vi "CAlex2_SetCuff_Thigh_Treadmill.vi"(9 "Extra Weight (kg)":dbl, 10 "Upper Cuff to Lower Cuff (m)":dbl, 11 "Lower Cuff to Knee (m)":dbl) -> (2 "Thigh Cuff Low":T1={"BodyID"=0, "CoM(CuffCS)"={"Coord4"=[0.0, 0.0, 0.0, 1.0], "ID"=0}, "Mass(kg)"=0.0, "CablePts(CuffCS)"=[], "Cuff->Body"=[[1.0, 0.0, 0.0, 0.0], [0.0, 1.0, 0.0, 0.0], [0.0, 0.0, 1.0, 0.0], [0.0, 0.0, 0.0, 1.0]]}, 3 "Thigh Cuff High":T1={"BodyID"=0, "CoM(CuffCS)"={"Coord4"=[0.0, 0.0, 0.0, 1.0], "ID"=0}, "Mass(kg)"=0.0, "CablePts(CuffCS)"=[], "Cuff->Body"=[[1.0, 0.0, 0.0, 0.0], [0.0, 1.0, 0.0, 0.0], [0.0, 0.0, 1.0, 0.0], [0.0, 0.0, 0.0, 1.0]]})   [LabVIEW 2016, in "CAlex2.lvclass"]
uses:
  CAlex2.lvclass
  SerialChain-Cable/TypeDef/Cuff.ctl
  SerialChain/TypeDef/PointOnBody.ctl
  <vilib>/Analysis/Matrix/Datatypes/RealMatrix.ctl
  SerialChain/TypeDef/xyzO.ctl
  <vilib>/Analysis/Matrix/NI_Matrix.lvlib
  SerialChain/SerialChain.lvclass
  SerialChain-Cable/SerialChain-Cable.lvclass
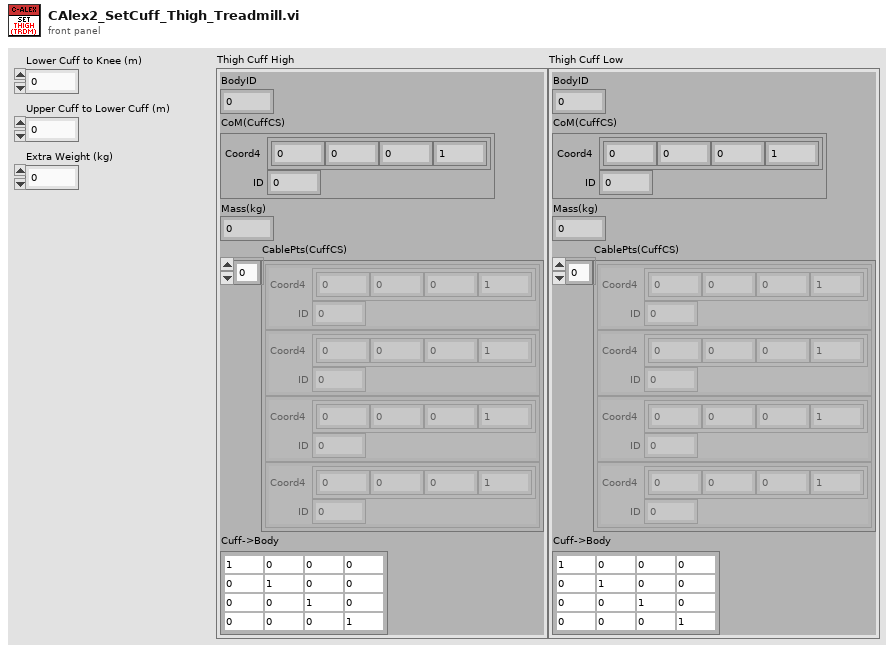
[diagram p1: front panel]
types:
  T1 = typedef "SerialChain-Cable.lvclass/Cuff.ctl" = cluster{"BodyID":i32, "CoM(CuffCS)":T2, "Mass(kg)":dbl, "CablePts(CuffCS)":T2[], "Cuff->Body":T3}
  T2 = typedef "SerialChain.lvclass/PointOnBody.ctl" = cluster{"Coord4":dbl[], "ID":i32}
  T3 = typedef "NI_Matrix.lvlib/RealMatrix.ctl" = dbl[][]
  T4 = typedef "SerialChain.lvclass/xyzO.ctl" = enum16{"X", "Y", "Z", "O"}
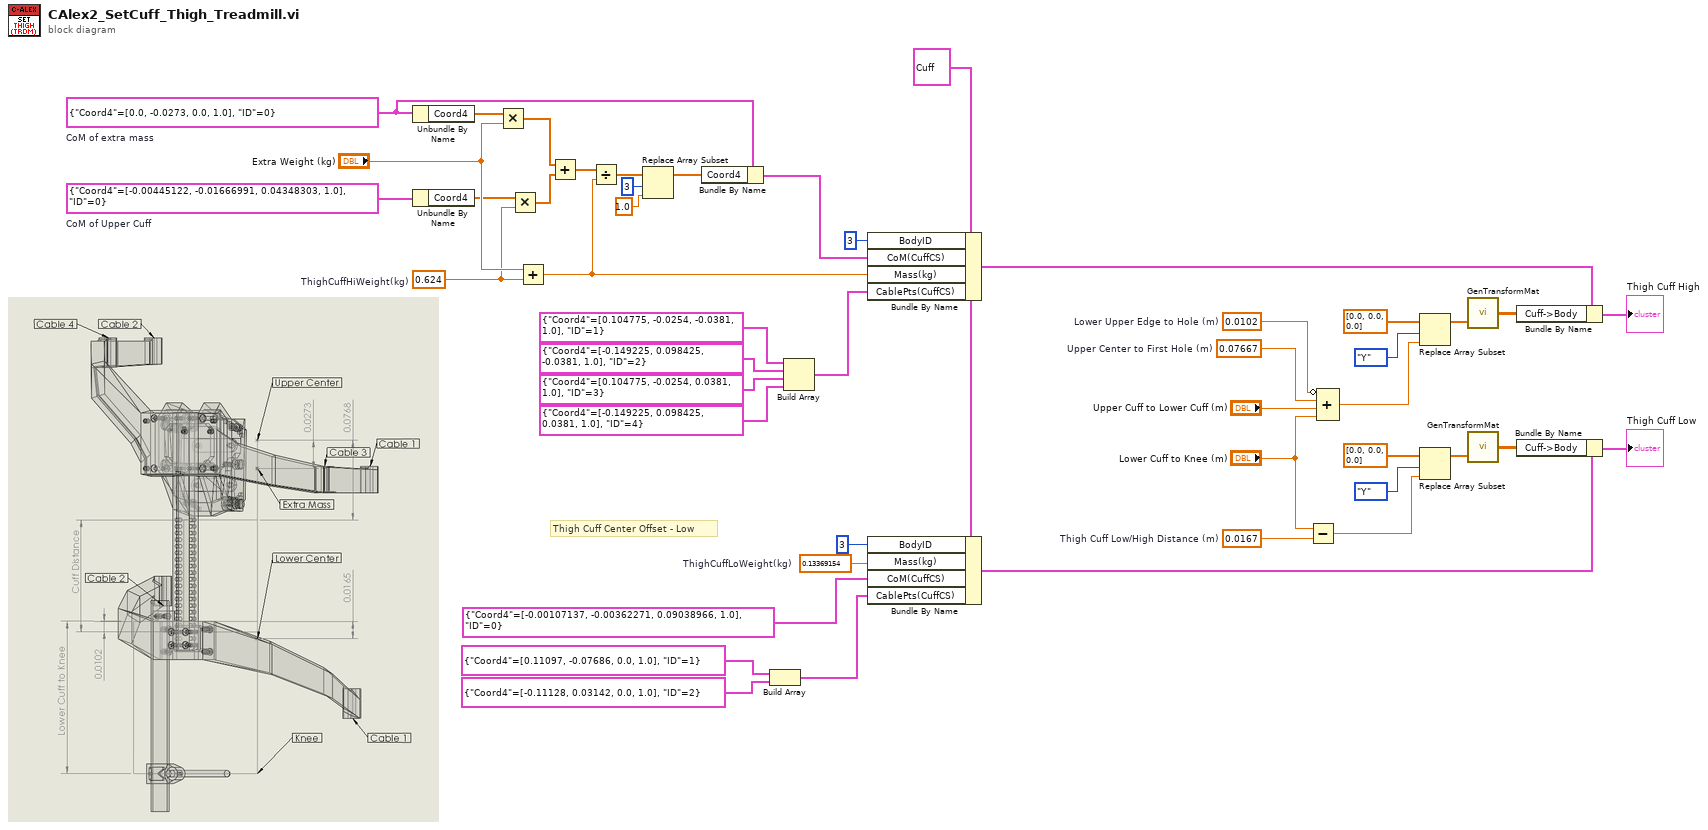
[diagram p0: block diagram]
diagram:
  w9 = 0.07667  # Upper Center to First Hole (m)
  w2 = 0.0102  # Lower Upper Edge to Hole (m)
  w17 = 0.0167  # Thigh Cuff Low/High Distance (m)
  w27 = T2 {"Coord4"=[0.0, -0.0273, 0.0, 1.0], "ID"=0}  # CoM of extra mass
  w38 = 0.13369154  # ThighCuffLoWeight(kg)
  w32 = 0.624  # ThighCuffHiWeight(kg)
  w36 = T2 {"Coord4"=[-0.00445122, -0.01666991, 0.04348303, 1.0], "ID"=0}  # CoM of Upper Cuff
  w20 = T1 {"BodyID"=0, "CoM(CuffCS)"={"Coord4"=[0.0, 0.0, 0.0, 1.0], "ID"=0}, "Mass(kg)"=0.0, "CablePts(CuffCS)"=[], "Cuff->Body"=[[1.0, 0.0, 0.0, 0.0], [0.0, 1.0, 0.0, 0.0], [0.0, 0.0, 1.0, 0.0], [0.0, 0.0, 0.0, 1.0]]} ("Cuff Design")
  # "Thigh Cuff Center Offset - Low"
  n1 = Unbundle By Name(w27) -> ("Coord4"=w35:dbl[])
  n2 = Unbundle By Name(w36) -> ("Coord4"=w33:dbl[])
  n3 = Multiply(x=w35, y="Extra Weight (kg)") -> (x*y=w31:dbl[])
  n4 = Multiply(x=w33, y=w32) -> (x*y=w30:dbl[])
  n5 = Add(x="Extra Weight (kg)", y=w32) -> (x+y=w28:dbl)
  n6 = Add(x=w31, y=w30) -> (x+y=w29:dbl[])
  n7 = Divide(x=w29, y=w28) -> (x/y=w25:dbl[])
  n8 = Replace Array Subset(array=w25, new element=1.0 ("new element/subarray"), index=3) -> (w24:dbl[])
  n9 = Bundle By Name(cluster=w27, "Coord4"=w24) -> (w26:T2)
  n10 = Build Array(T2 {"Coord4"=[0.11097, -0.07686, 0.0, 1.0], "ID"=1} ("CoM(CuffCS)"), T2 {"Coord4"=[-0.11128, 0.03142, 0.0, 1.0], "ID"=2} ("CoM(CuffCS)")) -> (w39:T2[])
  n11 = Build Array(T2 {"Coord4"=[0.104775, -0.0254, -0.0381, 1.0], "ID"=1} ("CoM(CuffCS)"), T2 {"Coord4"=[-0.149225, 0.098425, -0.0381, 1.0], "ID"=2} ("CoM(CuffCS)"), T2 {"Coord4"=[0.104775, -0.0254, 0.0381, 1.0], "ID"=3} ("CoM(CuffCS)"), T2 {"Coord4"=[-0.149225, 0.098425, 0.0381, 1.0], "ID"=4} ("CoM(CuffCS)")) -> (w44:T2[])
  n12 = Bundle By Name(cluster=w20, "BodyID"=3, "CoM(CuffCS)"=w26, "Mass(kg)"=w28, "CablePts(CuffCS)"=w44) -> (w18:T1)
  n13 = Bundle By Name(cluster=w20, "BodyID"=3, "Mass(kg)"=w38, "CoM(CuffCS)"=T2 {"Coord4"=[-0.00107137, -0.00362271, 0.09038966, 1.0], "ID"=0}, "CablePts(CuffCS)"=w39) -> (w19:T1)
  n14 = Subtract(x="Lower Cuff to Knee (m)", y=w17) -> (x-y=w11:dbl)
  n15 = Compound Arithmetic op=ADD(invert w2, w9, "Upper Cuff to Lower Cuff (m)", "Lower Cuff to Knee (m)") -> (w6:dbl)
  n16 = Replace Array Subset(array=dbl[] [0.0, 0.0, 0.0], new element=w6, index=xyzO."Y" ("XYZ")) -> (w5:dbl[])
  n17 = Replace Array Subset(array=dbl[] [0.0, 0.0, 0.0], new element=w11, index=xyzO."Y" ("XYZ")) -> (w13:dbl[])
  n18 = call "GenTransformMat.vi"("Translate 3Vector"=w5) -> ("Transformation Matrix"=w4:T3)  [unwired: 1 in]
  n19 = call "GenTransformMat.vi"("Translate 3Vector"=w13) -> ("Transformation Matrix"=w15:T3)  [unwired: 1 in]
  n20 = Bundle By Name(cluster=w18, "Cuff->Body"=w4) -> (→"Thigh Cuff High":T1)
  n21 = Bundle By Name(cluster=w19, "Cuff->Body"=w15) -> (→"Thigh Cuff Low":T1)
